vi "Read Data.vi"(8 "error in (no error)":errorcluster, 10 "Count":i32, 11 "StringStream in":refnum<class "StringStream.lvclass">) -> (0 "error out":errorcluster, 2 "Data":string, 3 "StringStream out":refnum<class "StringStream.lvclass">)   [LabVIEW 2020, in "IO.lvlib" / "StringStream.lvclass"]
uses:
  StringStream.lvclass
  StringStream.lvclass/StringStream.ctl
  <vilib>/Utility/error.llb/Error Cluster From Error Code.vi
  <vilib>/ErrorRing/Error Ring.xnode
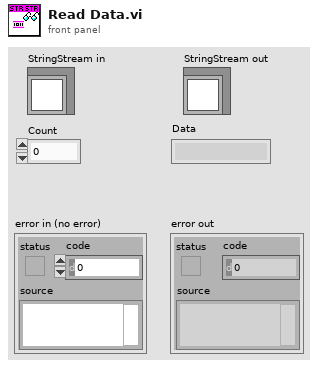
[diagram p1: front panel]
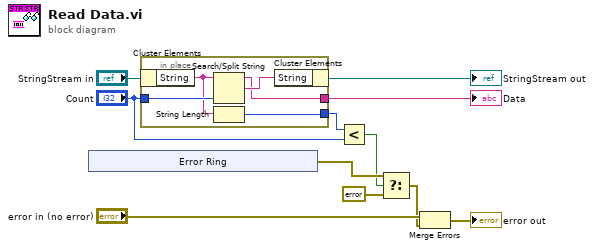
[diagram p0: block diagram]
diagram:
  n1 = xnode ("Error Ring")() -> ("error out"=w7:errorcluster)
  n2 = in-place "In Place Element Structure" {
    in-place-border: "Count" -> [w16]
    in-place-border: [w14] -> w11
    in-place-border: [w12] -> w9
    n3 = in-place-cluster #1("StringStream in") -> ("String"=w13:string)
    n4 = Search/Split String(string=w13, offset (0)=w16) -> (substring before match=w14:string, match + rest of string=w15:string)  [unwired: 1 in, 1 out]
    n5 = String Length(string=w13) -> (length=w12:i32)
    n6 = in-place-cluster #1("String"=w15) -> (→"StringStream out":refnum<class "StringStream.lvclass">)
  }
  "Data" <- w11
  n7 = Less?(x=w9, y="Count") -> (x < y?=w5:bool)
  n8 = Select(t=w7, s=w5, f=errorcluster {"status"=FALSE, "code"=0, "source"=""}) -> (s? t:f=w3:errorcluster)
  n9 = Merge Errors("error in (no error)", w3) -> (→"error out":errorcluster)
